vi "Process Command.vi"(4 "error in (no error)":errorcluster, 7 "Set TC Params in":refnum<class "Remote Access Commands_Set TC Parameters.lvclass">) -> (0 "error out":errorcluster, 2 "Response out":T1, 3 "Set TC Params out":refnum<class "Remote Access Commands_Set TC Parameters.lvclass">)   [LabVIEW 2015, in "Startup Processes.lvlib" / "Remote Access Commands_Set TC Parameters.lvclass"]
uses:
  Remote Access Commands_Set TC Parameters.lvclass
  _typedefs/JSON Response Cluster.ctl
  _typedefs/Custom Remote Access Error Codes.ctl
  Toolbox/Standard Signalling/not_Generic Named Notifier/not_Generic Named Notifier.lvlib
  Remote Access Commands.lvclass
  Startup Processes.lvlib
  _ude/Set TC Parameters/Set TC Parameters.lvlib
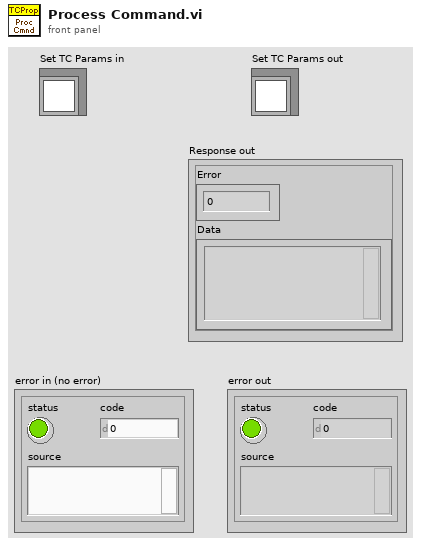
[diagram p1: front panel]
types:
  T1 = typedef "Startup Processes.lvlib/JSON Response Cluster.ctl" = cluster{"Error":i32, "Data":string}
  T2 = typedef "Startup Processes.lvlib/Custom Remote Access Error Codes.ctl" = enum16{"No Error", "CRC Error", "Update Failed"}
  T3 = typedef "Startup Processes.lvlib/TC Setup Parameters.ctl" = cluster{"Error High Level":dbl, "Warning High Level":dbl, "Warning Low Level":dbl, "Error Low Level":dbl, "Sample Interval":dbl[unit]}
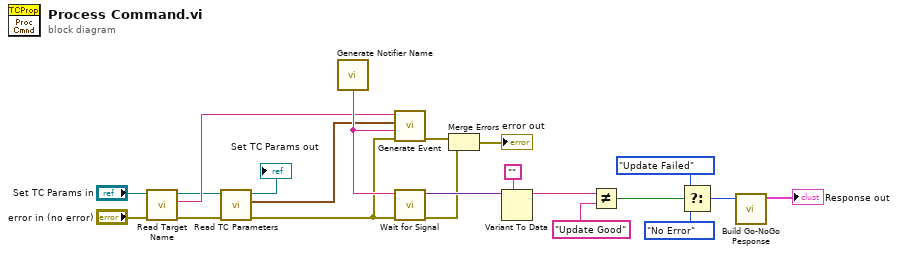
[diagram p0: block diagram]
diagram:
  n1 = call "Read Target Name.vi"("Error In"="error in (no error)", "Remote Access Commands in"="Set TC Params in") -> ("Error Out"=w9:errorcluster, "Target Name"=w16:string, "Remote Access Commands out"=w11:refnum<class "Remote Access Commands_Set TC Parameters.lvclass">)  [unwired: 3 in]
  n2 = call-dynamic "Read TC Parameters.vi"("Error In"=w9, "Set TC Parameters in"=w11) -> ("Error Out"=w8:errorcluster, "TC Parameters"=w1:T3, "Set TC Parameters out"=→"Set TC Params out":refnum<class "Remote Access Commands_Set TC Parameters.lvclass">)  [unwired: 3 in]
  n3 = call "Generate Notifier Name.vi"() -> ("Notifier Name"=w20:string)
  n4 = call "Generate Event.vi"("Error In"=w8, "Response Notifier"=w20, "TC Parameters"=w1, "Plugin Name"=w16) -> ("Error Out"=w21:errorcluster)  [unwired: 3 in]
  n5 = call "Wait for Signal.vi"("Error In"=w8, "Notifier Name"=w20) -> ("Error Out"=w12:errorcluster, "Signal Data"=w15:variant)  [unwired: 4 in]
  n6 = Merge Errors(w21, w12) -> (→"error out":errorcluster)
  n7 = Variant To Data(type="", Variant=w15) -> (data=w4:string)  [unwired: 1 in, 1 out]
  n8 = Not Equal?(x=w4, y="Update Good") -> (x != y?=w3:bool)
  n9 = Select(t=Custom_Remote_Access_Error_Codes."Update Failed" ("Error"), s=w3, f=Custom_Remote_Access_Error_Codes."No Error" ("Error")) -> (s? t:f=w5:T2)
  n10 = call "Build Go-NoGo Pesponse.vi"("Error"=w5) -> ("Response"=→"Response out":T1)  [unwired: 5 in, 1 out]
